vi "Submit.vi"(0 "Commit in":refnum<class "Commit.lvclass">, 5 "Export":refnum<class "Export.lvclass">, 11 "error in (no error)":errorcluster) -> (4 "Commit out":refnum<class "Commit.lvclass">, 15 "error out":errorcluster)   [LabVIEW 2017, in "CL_G3_VIComponentBuilder.lvlib" / "Commit.lvclass"]
doc: "Performs the submit operations for this export."
uses:
  Commit.lvclass
  Exports/Exports/Export.lvclass
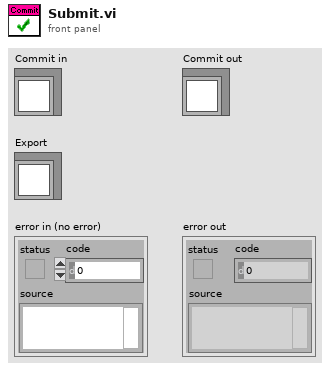
[diagram p1: front panel]
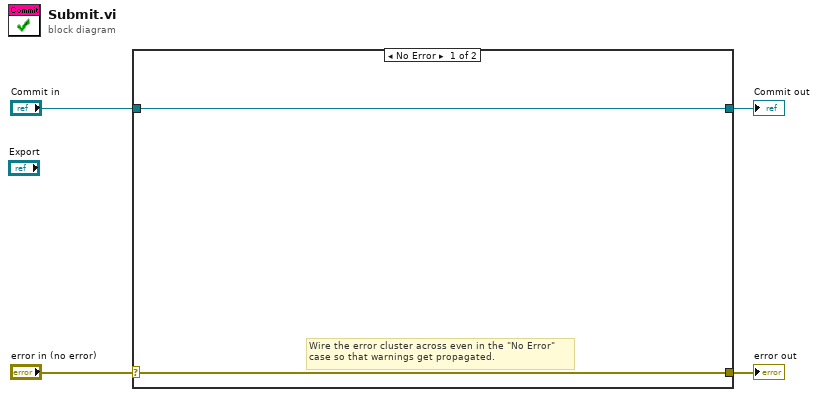
[diagram p0: block diagram]
diagram:
  n1 = case shown="No Error" "error in (no error)" {
    selector: "error in (no error)" -> [w6 w8]
    tunnel: [w6 w8] -> w3
    tunnel: [w5 w7] -> w1
    tunnel: "Commit in" -> [w5 w7]
    frame No Error {
      # "Wire the error cluster across even in the \"No Error\"\ncase so that warnings get propagated."
    }
    frame Error {
    }
  }
  "error out" <- w3
  "Commit out" <- w1
